vi "_PC_NS_Wfm_Init_Status.vi"(5 "wfm stop bool":refnum<k21>, 7 "wfm connect status":refnum<k21>, 8 "error IO":errorcluster) -> (0 "error Out":errorcluster)   [LabVIEW 2018]
uses:
  RT/PublicSubVI/Ctl/_ctl_RT_NS_Status.ctl
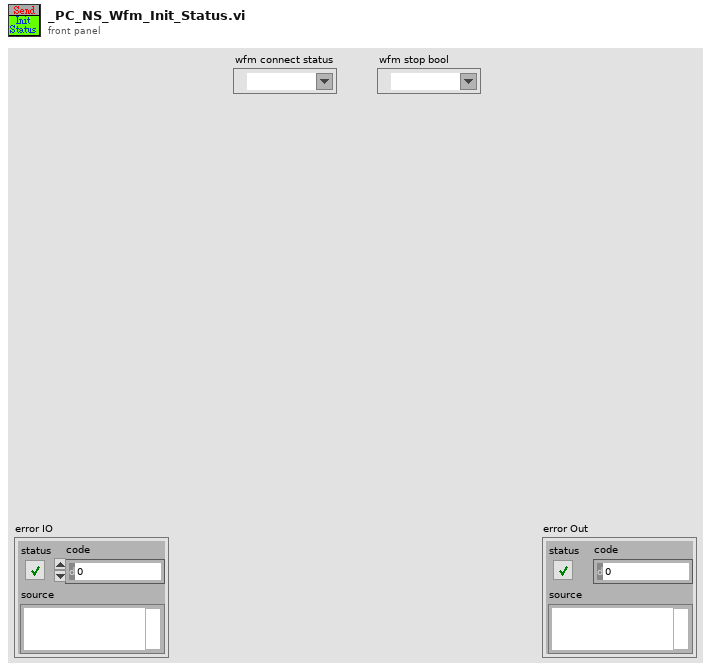
[diagram p1: front panel]
types:
  T1 = typedef "_ctl_RT_NS_Status.ctl" = enum8{"Idle", "Init", "Connected", "Stop"}
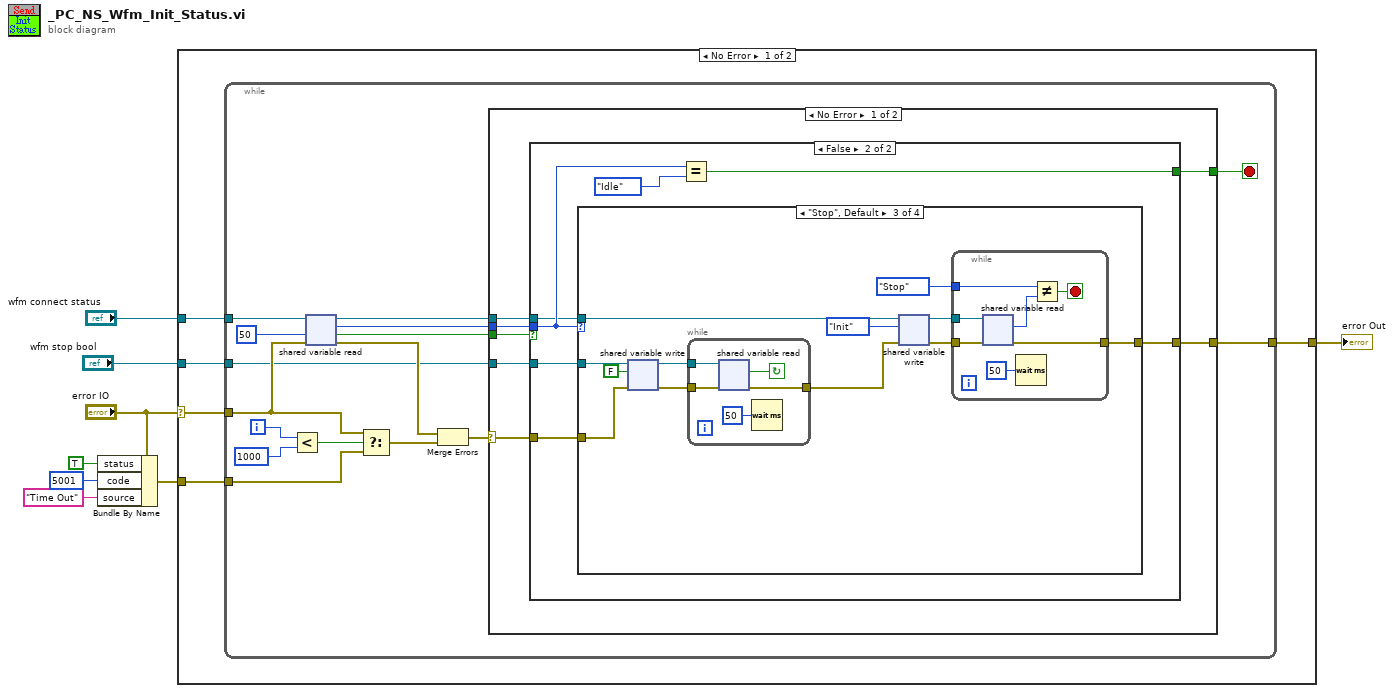
[diagram p0: block diagram]
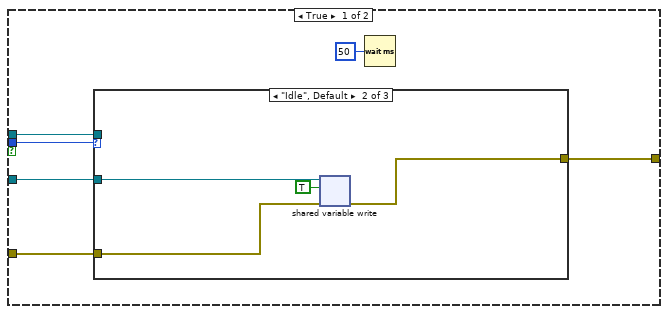
[diagram p2: hidden frame]
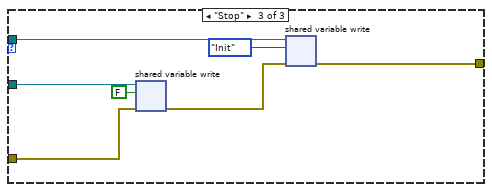
[diagram p4: hidden frame]
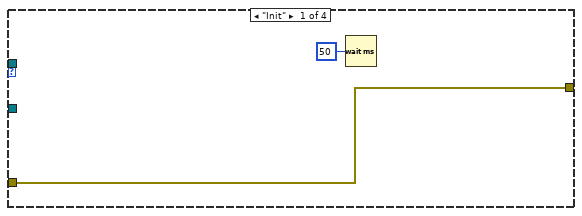
[diagram p5: hidden frame]
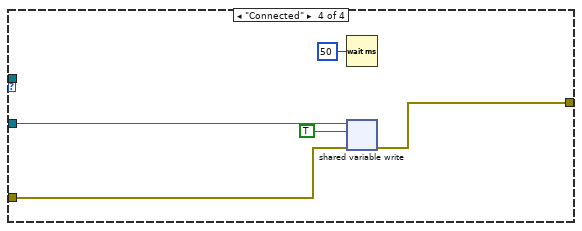
[diagram p7: hidden frame]
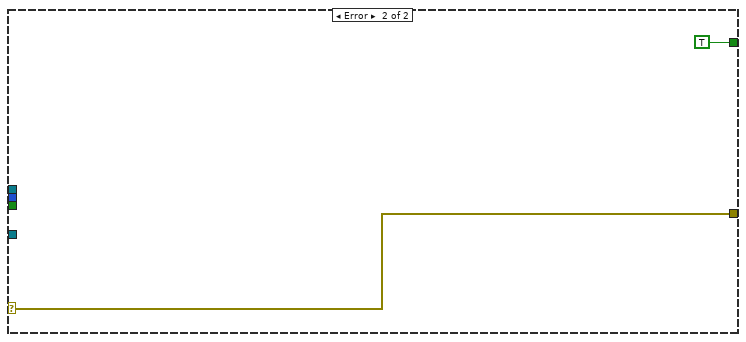
[diagram p8: hidden frame]
diagram:
  n1 = Bundle By Name(cluster="error IO", "status"=TRUE, "code"=5001, "source"="Time Out") -> (w6:errorcluster)
  n2 = case shown="No Error" "error IO" {
    selector: "error IO" -> [w9 w96]
    tunnel: [w13 w96] -> w8
    tunnel: w6 -> [w12 _]
    tunnel: "wfm connect status" -> [w11 _]
    tunnel: "wfm stop bool" -> [w10 _]
    frame No Error {
      n3 = while {
        tunnel: w12 -> [w23]
        tunnel: w11 -> [w21]
        tunnel: w10 -> [w15]
        tunnel: [w29] -> w13
        tunnel: w9 -> [w16]
        i -> [w26]
        stop <- w28 stop-if-true
        n4 = Less?(x=w26, y=1000) -> (x < y?=w24:bool)
        n5 = shared-variable-read(w21, w16, 50 ("ms timeout (0)")) -> (w14:refnum<k21>, w17:errorcluster, w18:bool, w19:T1)  [unwired: 1 out]
        n6 = Select(t=w16, s=w24, f=w23) -> (s? t:f=w22:errorcluster)
        n7 = Merge Errors(w17, w22) -> (w27:errorcluster)
        n8 = case shown="No Error" w27 {
          selector: w27 -> [w32 w94]
          tunnel: [w36 w94] -> w29
          tunnel: [w35 TRUE] -> w28
          tunnel: w19 -> [w34 _]
          tunnel: w18 -> [w33 _]
          tunnel: w15 -> [w31 _]
          tunnel: w14 -> [w30 _]
          frame No Error {
            n9 = case shown="False" w33 {
              tunnel: w34 -> [w41 w60]
              tunnel: [w40 w59] -> w36
              tunnel: w32 -> [w39 w58]
              tunnel: [_ w57] -> w35
              tunnel: w31 -> [w38 w55]
              tunnel: w30 -> [w37 w56]
              frame True {
                n10 = case shown="\"Idle\", Default" w41 {
                  tunnel: [w43 w44 w48] -> w40
                  tunnel: w39 -> [w43 w45 w53]
                  tunnel: w38 -> [_ w46 w52]
                  tunnel: w37 -> [_ _ w51]
                  frame "Init" {
                  }
                  frame "Idle", Default {
                    n11 = shared-variable-write(w46, w45, TRUE ("data in")) -> (w44:errorcluster)  [unwired: 1 out]
                  }
                  frame "Stop" {
                    n12 = shared-variable-write(w52, w53, FALSE ("data in")) -> (w50:errorcluster)  [unwired: 1 out]
                    n13 = shared-variable-write(w51, w50, _ctl_RT_NS_Status."Init" ("Wfm_Connect_Status")) -> (w48:errorcluster)  [unwired: 1 out]
                  }
                }
                n14 = Wait (ms)(milliseconds to wait=u32 50) -> ()  [unwired: 1 out]
              }
              frame False {
                n15 = case shown="\"Stop\", Default" w60 {
                  tunnel: w58 -> [w63 w64 w73 w90]
                  tunnel: [w63 w64 w65 w89] -> w59
                  tunnel: w56 -> [_ _ w69 _]
                  tunnel: w55 -> [_ _ w76 w92]
                  frame "Init" {
                    n16 = Wait (ms)(milliseconds to wait=u32 50) -> ()  [unwired: 1 out]
                  }
                  frame "Idle" {
                  }
                  frame "Stop", Default {
                    n17 = shared-variable-write(w76, w73, FALSE ("data in")) -> (w72:refnum<k21>, w74:errorcluster)
                    n18 = while {
                      tunnel: w74 -> [w88]
                      tunnel: w72 -> [w86]
                      tunnel: [w84] -> w68
                      stop <- w85 continue-if-true
                      n19 = shared-variable-read(w86, w88) -> (w84:errorcluster, w85:bool)  [unwired: 1 out]
                      n20 = Wait (ms)(milliseconds to wait=u32 50) -> ()  [unwired: 1 out]
                    }
                    n21 = shared-variable-write(w69, w68, _ctl_RT_NS_Status."Init" ("Signal_RT_Status")) -> (w70:refnum<k21>, w71:errorcluster)
                    n22 = while {
                      tunnel: w71 -> [w83]
                      tunnel: w70 -> [w81]
                      tunnel: [w80] -> w65
                      tunnel: _ctl_RT_NS_Status."Stop" ("t") -> [w78]
                      stop <- w77 stop-if-true
                      n23 = shared-variable-read(w81, w83) -> (w80:errorcluster, w79:T1)  [unwired: 2 out]
                      n24 = Wait (ms)(milliseconds to wait=u32 50) -> ()  [unwired: 1 out]
                      n25 = Not Equal?(x=w78, y=w79) -> (x != y?=w77:bool)
                    }
                  }
                  frame "Connected" {
                    n26 = Wait (ms)(milliseconds to wait=u32 50) -> ()  [unwired: 1 out]
                    n27 = shared-variable-write(w92, w90, TRUE ("Signal_Stop_Bool")) -> (w89:errorcluster)  [unwired: 1 out]
                  }
                }
                n28 = Equal?(x=w60, y=_ctl_RT_NS_Status."Idle") -> (x = y?=w57:bool)
              }
            }
          }
          frame Error {
          }
        }
      }
    }
    frame Error {
    }
  }
  "error Out" <- w8
